vi "AVS_go_Remote.vi"(3 "Timeout (sec)":i16=1 min=0 max=3600 step=1, 4 "VISA-AVS":refnum<visa-resource-name>) -> (0 "error out":errorcluster, 1 "dup VISA session":refnum<visa-resource-name>)   [LabVIEW 2019]
panel:
  in  "error in (no error)":errorcluster
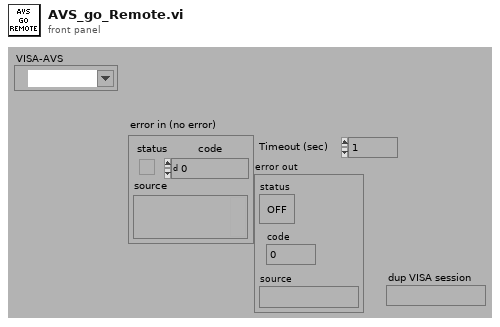
[diagram p1: front panel]
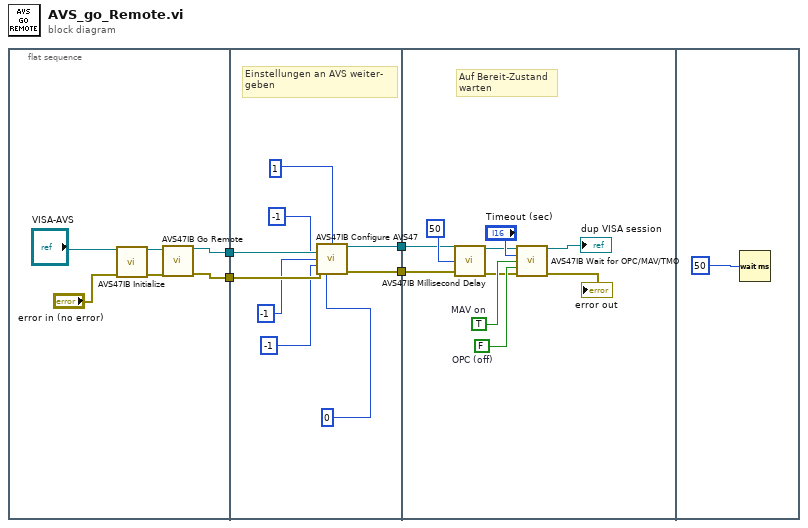
[diagram p0: block diagram]
diagram:
  n1 = flat-sequence {
    tunnel: [w7] -> w4
    tunnel: [w6] -> w3
    tunnel: w4 -> [w19]
    tunnel: w3 -> [w18]
    tunnel: [w17] -> w2
    tunnel: [w16] -> w1
    tunnel: w2 -> [w23]
    tunnel: w1 -> [w22]
    frame #0 {
      n2 = call "AVS47IB Initialize.vi"("VISA session (for class)"="VISA-AVS", "error in (no error)"="error in (no error)") -> ("VISA session"=w9:refnum<visa-resource-name>, "error out"=w8:errorcluster)  [unwired: 12 in]
      n3 = call "AVS47IB Go Remote.vi"("VISA session"=w9, "error in (no error)"=w8) -> ("dup VISA session"=w7:refnum<visa-resource-name>, "error out"=w6:errorcluster)  [unwired: 12 in]
    }
    frame #1 {
      # "Einstellungen an AVS weiter-\ngeben"
      n4 = call "AVS47IB Configure AVS47.vi"("VISA session"=w19, "INPUT (-1:no change)"=i8 1, "CHANNEL (-1:no change )"=i8 -1, "RANGE  (-1:no change)"=i8 -1, "EXCITATION (-1:no change)"=i8 -1, "error in (no error)"=w18, "DISPLAY (-1:no change)"=i8 0) -> ("dup VISA session"=w17:refnum<visa-resource-name>, "error out"=w16:errorcluster)  [unwired: 7 in]
    }
    frame #2 {
      w28 = FALSE  # OPC (off)
      w29 = TRUE  # MAV on
      # "Auf Bereit-Zustand\nwarten"
      n5 = call "AVS47IB Millisecond Delay.vi"("VISA session"=w23, "Delay (50 ms)"=u32 50, "error in (no error)"=w22) -> ("dup VISA session"=w26:refnum<visa-resource-name>, "error out"=w25:errorcluster)  [unwired: 11 in]
      n6 = call "AVS47IB Wait for OPC/MAV/TMO.vi"("VISA session"=w26, "Timeout (2 sec)"="Timeout (sec)", "MAV (on)"=w29, "OPC (off)"=w28, "error in (no error)"=w25) -> ("dup VISA session"=→"dup VISA session":refnum<visa-resource-name>, "error out"=→"error out":errorcluster)  [unwired: 8 in, 1 out]
    }
    frame #3 {
      n7 = Wait (ms)(milliseconds to wait=50) -> ()  [unwired: 1 out]
    }
  }
